vi "calibMagnetometersSetTransformations.vi"(8 "error in (no error)":errorcluster, 9 "crossAxis":sgl[](array[numeric])=[0.0, 0.0, 0.0, 0.0, 0.0, 0.0, 0.0, 0.0, 0.0], 10 "offset":sgl[](array[numeric])=[0.0, 0.0, 0.0], 11 "pHandle":u32) -> (0 "error out":errorcluster, 3 "return type":i32)   [LabVIEW 2011, in "sbgLabView.lvlib"]
uses:
  sbgLabView.lvlib
  sbgMatLab.dll
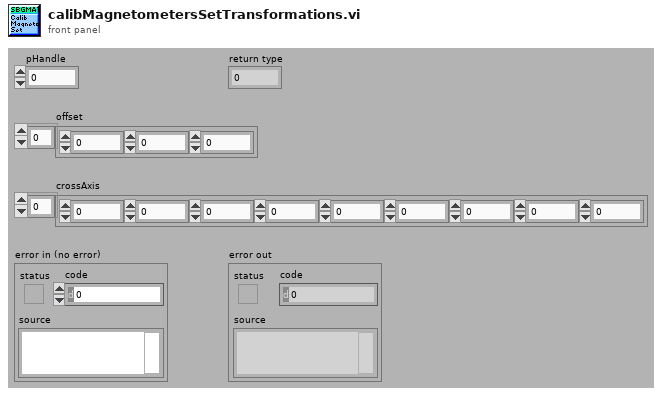
[diagram p1: front panel]
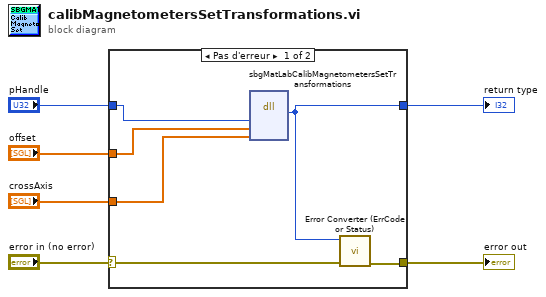
[diagram p0: block diagram]
diagram:
  n1 = case shown="Pas d'erreur" "error in (no error)" {
    selector: "error in (no error)" -> [w8 w13]
    tunnel: [w7 w13] -> w5
    tunnel: [w12 _] -> w4
    tunnel: "pHandle" -> [w11 _]
    tunnel: "offset" -> [w10 _]
    tunnel: "crossAxis" -> [w9 _]
    frame No Error {
      n2 = dll-call lib="C:/SBG-Systems/remote/projects/software/projects/labviewExample/sbgLabView/sbgMatLab.*" fn="sbgMatLabCalibMagnetometersSetTransformations"("pHandle"=w11, "offset"=w10, "crossAxis"=w9) -> ("return type"=w12:i32)  [unwired: 6 in, 2 out]
      n3 = call "Error Converter (ErrCode or Status).vi"("error in (no error)"=w8, "error code"=w12) -> ("error out"=w7:errorcluster)  [unwired: 9 in]
    }
    frame Error {
    }
  }
  "return type" <- w4
  "error out" <- w5
